vi "Test Complete Core.vi"(8 "Vehicle":string, 9 "SMS Recipients":u32, 11 "File Name":string) -> ()   [LabVIEW 2014]
panel:
  out "Boolean array":bool[](array[boolean])
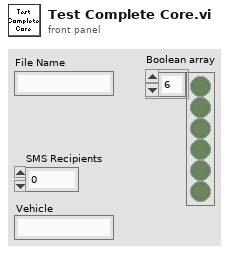
[diagram p1: front panel]
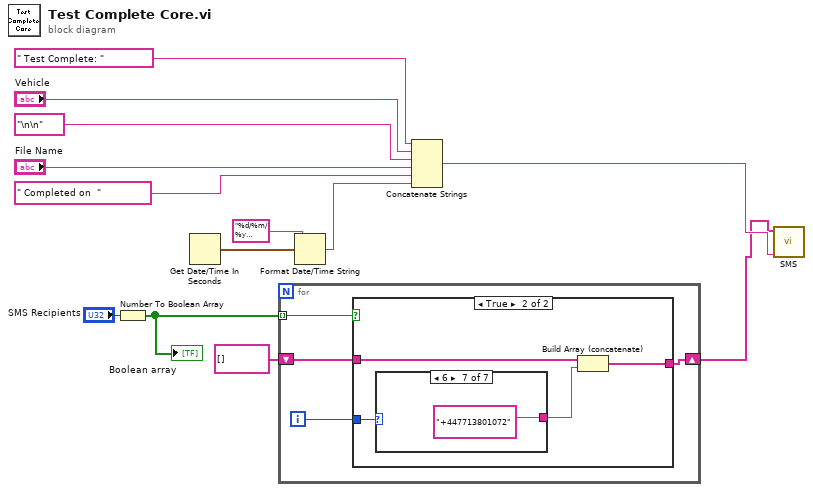
[diagram p0: block diagram]
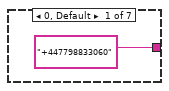
[diagram p3: hidden frame]
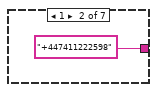
[diagram p4: hidden frame]
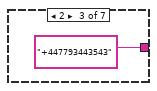
[diagram p5: hidden frame]
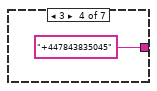
[diagram p6: hidden frame]
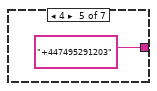
[diagram p7: hidden frame]
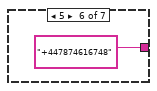
[diagram p8: hidden frame]
diagram:
  n1 = Number To Boolean Array(number="SMS Recipients") -> (Boolean array=w12:bool[])
  "Boolean array" <- w12
  n2 = Get Date/Time In Seconds() -> (seconds since 1Jan1904=w10:timestamp)
  n3 = for {
    tunnel: w12 -> [w17] mode=indexing
    shift-right: [w14] -> w1
    shift-left: string[] [] -> [w15]
    i -> [w16]
    n4 = case shown="True" w17 {
      tunnel: w16 -> [_ w22]
      tunnel: w15 -> [w18 w21]
      tunnel: [w18 w19] -> w14
      frame False {
      }
      frame True {
        n5 = case shown="6" w22 {
          tunnel: ["+447798833060" ("String") "+447411222598" ("String") "+447793443543" ("String") "+447843835045" ("String") "+447495291203" ("String") "+447874616748" ("String") "+447713801072" ("String")] -> w20
          frame 0, Default {
          }
          frame 1 {
          }
          frame 2 {
          }
          frame 3 {
          }
          frame 4 {
          }
          frame 5 {
          }
          frame 6 {
          }
        }
        n6 = Build Array (concatenate)(w21, w20) -> (w19:string[])
      }
    }
  }
  n7 = Format Date/Time String(time format string (%c)="%d/%m/%y %H:%M:%S", seconds (now)=w10) -> (date/time string=w7:string)  [unwired: 1 in]
  n8 = Concatenate Strings(" Test Complete: " ("string"), "Vehicle", "\n\n" ("string"), "File Name", " Completed on  " ("string"), w7) -> (w2:string)
  n9 = call "SMS.vi"("text"=w2, "phoneNumbers"=w1) -> ()  [unwired: 10 in]
